vi "SendPlotInfoAsJSON.vi"(0 "reference in":refnum<class "HTMLPlot.lvclass">, 2 "PlotInfo":variant, 5 "error in (no error)":errorcluster) -> (14 "reference out":refnum<class "HTMLPlot.lvclass">, 19 "error out":errorcluster)   [LabVIEW 2019, in "HTMLPlot.lvclass"]
uses:
  HTMLPlot.lvclass
  9a1ee0f5-a3c5-401c-b70f-fbea9e6d419a.vi
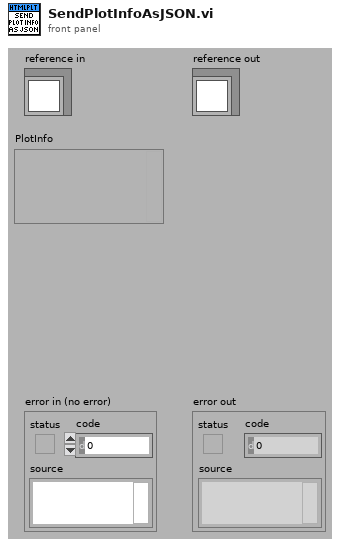
[diagram p1: front panel]
types:
  T1 = enum16{"Standard", "Buffered", "CRLF", "Immediate"}
  T2 = typedef "HTMLPlot.lvclass/ObjectAttributes.ctl" = cluster{"Attribute1":dbl, "GraphContainer":refnum<k7>, "ChartScriptFile":string, "UtilScriptFile(demoData)":string, "BaseHTML":string, "GenericProperties":cluster{"PlotType":T3, "PlotTitle":string, "XLabel":string, "YLabel":string, "ShowToolTip":bool}, "LegendProperties":cluster{"Show":bool, "Position":T4}, "BarPlot":cluster{"Dataset":dbl[][], "DatasetLabels":string[], "XLabels":string[], "PlotColours":u32[], "Stacked":bool}, "PiePlot":cluster{"Dataset":dbl[][], "DatasetLabels":string[], "PlotColours":u32[], "DoughnutStyle":bool, "PlotLabels":string[]}, "connection ID":refnum<k5>, "PortID":u64}
  T3 = typedef "HTMLPlot.lvclass/PlotType.ctl" = enum16{"bar", "line", "pie"}
  T4 = typedef "HTMLPlot.lvclass/LegendPosition.ctl" = enum16{"top", "right", "left", "bottom"}
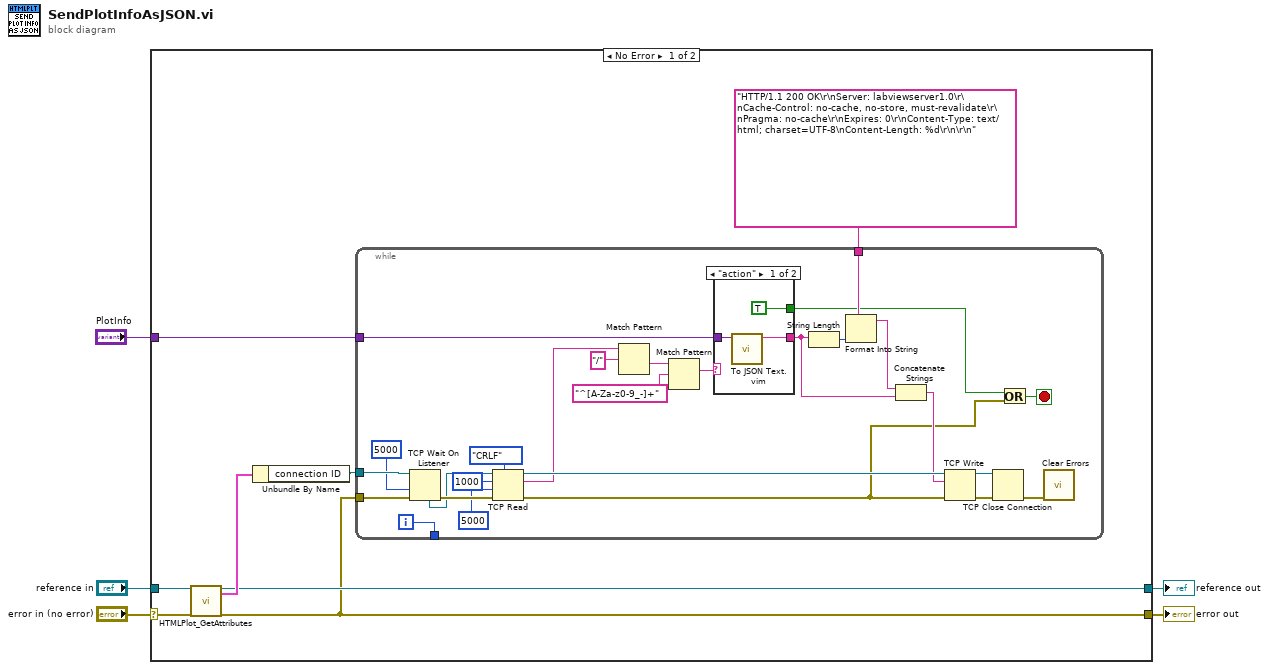
[diagram p0: block diagram]
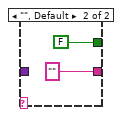
[diagram p2: hidden frame]
diagram:
  n1 = case shown="No Error" "error in (no error)" {
    selector: "error in (no error)" -> [w13 w47]
    tunnel: [w7 w47] -> w4
    tunnel: [w10 w46] -> w2
    tunnel: "reference in" -> [w12 w46]
    tunnel: "PlotInfo" -> [w6 _]
    frame No Error {
      n2 = call "HTMLPlot_GetAttributes.vi"("reference in"=w12, "error in (no error)"=w13) -> ("reference out"=w10:refnum<class "HTMLPlot.lvclass">, "Data"=w11:T2, "error out"=w7:errorcluster)  [unwired: 14 in, 1 out]
      n3 = Unbundle By Name(w11) -> ("connection ID"=w8:refnum<k5>)
      n4 = while {
        tunnel: "HTTP/1.1 200 OK\r\nServer: labviewserver1.0\r\nCache-Control: no-cache, no-store, must-revalidate\r\nPragma: no-cache\r\nExpires: 0\r\nContent-Type: text/html; charset=UTF-8\nContent-Length: %d\r\n\r\n" ("headers") -> [w24]
        tunnel: w7 -> [w22]
        tunnel: w8 -> [w21]
        tunnel: [w20] -> _
        tunnel: w6 -> [w19]
        i -> [w20]
        stop <- w15 stop-if-true
        n5 = TCP Wait On Listener(8:w22, 9:5000 ("timeout ms (25000)"), 11:w21) -> (0:w35:errorcluster, 4:w34:refnum<k5>)  [unwired: 1 in, 3 out]
        n6 = TCP Read(connection ID=w34, bytes to read=1000, error in (no error)=w35, 7:T1."CRLF" ("mode (standard)"), 9:5000 ("timeout ms (25000)")) -> (connection ID out=w38:refnum<k5>, data out=w33:string, error out=w17:errorcluster)
        n7 = Match Pattern(string=w33, regular expression="/") -> (after substring=w31:string)  [unwired: 1 in, 3 out]
        n8 = Match Pattern(string=w31, regular expression="^[A-Za-z0-9_-]+") -> (match substring=w29:string)  [unwired: 1 in, 3 out]
        n9 = case shown="\"action\"" w29 {
          tunnel: [w43 "" ("<JSON>")] -> w25
          tunnel: [TRUE FALSE] -> w16
          tunnel: w19 -> [w41 _]
          frame "action" {
            n10 = call "To JSON Text.vim"("Anything"=w41) -> ("<JSON>"=w43:string)  [unwired: 9 in, 1 out]
          }
          frame "", Default {
          }
        }
        n11 = String Length(string=w25) -> (length=w27:i32)
        n12 = Format Into String(format string=w24, w27) -> (resulting string=w28:string)  [unwired: 2 in, 1 out]
        n13 = Concatenate Strings(w28, w25) -> (w26:string)
        n14 = TCP Write(connection ID=w38, data in=w26, error in (no error)=w17) -> (connection ID out=w36:refnum<k5>, error out=w37:errorcluster)  [unwired: 1 in, 1 out]
        n15 = TCP Close Connection(connection ID=w36, error in (no error)=w37) -> (error out=w23:errorcluster)  [unwired: 1 in, 1 out]
        n16 = Or(x=w16, y=w17) -> (x .or. y?=w15:bool)
        n17 = call <vilib>:"Clear Errors.vi"("error in (no error)"=w23) -> ()  [unwired: 5 in, 2 out]
      }
    }
    frame Error {
    }
  }
  "error out" <- w4
  "reference out" <- w2
